vi "load_scan.vi"(8 "error in":errorcluster, 10 "values in":dbl[](array[numeric]) format="%#_8p") -> (0 "error out":errorcluster, 2 "values out":dbl[](array[numeric]) format="%#_8p")   [LabVIEW 2017, in "tools.lvlib"]
uses:
  tools.lvlib
  <vilib>/Utility/file.llb/Read Delimited Spreadsheet (DBL).vi
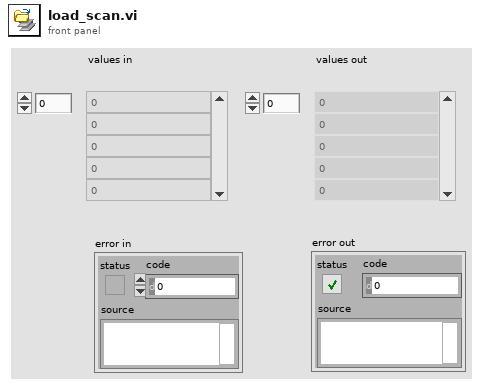
[diagram p1: front panel]
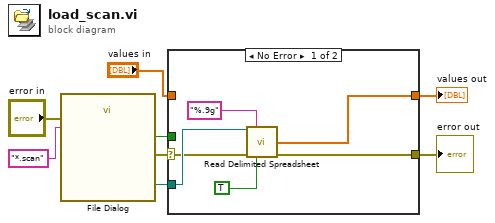
[diagram p0: block diagram]
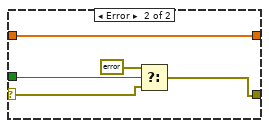
[diagram p2: hidden frame]
diagram:
  n1 = call "File Dialog"("error in"="error in", "pattern (all files)"="*.scan") -> ("selected path"=w7:path, "cancelled"=w1:bool, "error out"=w8:errorcluster)  [unwired: 10 in, 1 out]
  n2 = case shown="No Error" w8 {
    selector: w8 -> [w12 w17]
    tunnel: w7 -> [w13 _]
    tunnel: [w10 w19] -> w5
    tunnel: "values in" -> [_ w19]
    tunnel: [w9 w15] -> w2
    tunnel: w1 -> [_ w18]
    frame No Error {
      n3 = call-poly <vilib>:"Read Delimited Spreadsheet.vi"("file path (dialog if empty)"=w13, "format (%.3f)"="%.9g", "error in (no error)"=w12, "transpose? (F)"=TRUE) -> ("first row"=w10:dbl[], "error out"=w9:errorcluster)  [unwired: 6 in, 4 out]
    }
    frame Error {
      n4 = Select(t=errorcluster {"status"=FALSE, "code"=0, "source"=""}, s=w18, f=w17) -> (s? t:f=w15:errorcluster)
    }
  }
  "values out" <- w5
  "error out" <- w2
